vi "Feedforward.vi"(11 "Ref force":dbl) -> (3 "predict":dbl)   [LabVIEW 2021]
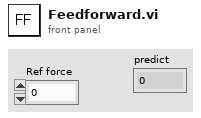
[diagram p1: front panel]
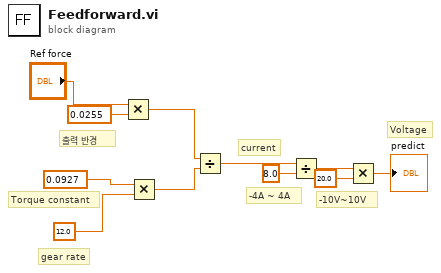
[diagram p0: block diagram]
diagram:
  # "Voltage"
  # "-10V~10V"
  # "-4A ~ 4A"
  # "current"
  # "Torque constant"
  # "gear rate"
  # "출력 반경"
  n1 = Multiply(x="Ref force", y=0.0255) -> (x*y=w9:dbl)
  n2 = Multiply(x=0.0927, y=12.0) -> (x*y=w6:dbl)
  n3 = Divide(x=w9, y=w6) -> (x/y=w5:dbl)
  n4 = Divide(x=w5, y=8.0) -> (x/y=w3:dbl)
  n5 = Multiply(x=w3, y=20.0) -> (x*y=→"predict":dbl)
